vi "GetCurrentPosition.vi"(8 "error in (no error)":errorcluster, 11 "Serial Controller in":refnum<class "Serial Controller.lvclass">) -> (0 "error out":errorcluster, 1 "PositionBundle":cluster{"X":dbl, "Y":dbl, "Z":dbl, "Depth":dbl}, 2 "Position":dbl[](array[numeric]), 3 "Serial Controller out":refnum<class "Serial Controller.lvclass">)   [LabVIEW 2012, in "Serial Controller.lvclass"]
uses:
  Serial Controller.lvclass
  Serial Controller.lvclass/Serial Controller.ctl
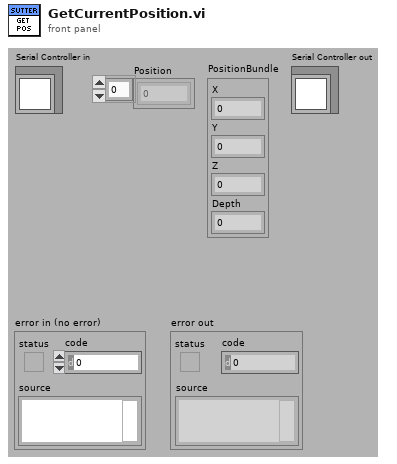
[diagram p1: front panel]
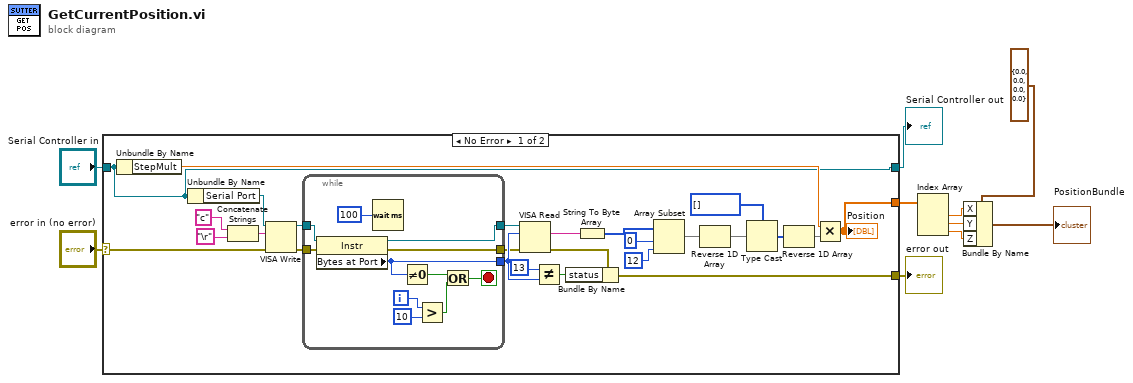
[diagram p0: block diagram]
diagram:
  n1 = case shown="No Error" "error in (no error)" {
    selector: "error in (no error)" -> [w16 w49]
    tunnel: [w12 w49] -> w3
    tunnel: [w26 w48] -> w9
    tunnel: "Serial Controller in" -> [w26 w48]
    tunnel: [w27 _] -> w7
    frame No Error {
      n2 = Unbundle By Name(w26) -> ("StepMult"=w28:dbl)
      n3 = Unbundle By Name(w26) -> ("Serial Port"=w20:refnum<visa-resource-name>)
      n4 = Concatenate Strings("c" ("string"), "\r" ("write buffer")) -> (w17:string)
      n5 = VISA Write(VISA resource name=w20, write buffer=w17, error in (no error)=w16) -> (VISA resource name out=w21:refnum<visa-resource-name>, error out=w15:errorcluster)  [unwired: 1 out]
      n6 = while {
        tunnel: w21 -> [w47]
        tunnel: w15 -> [w46]
        tunnel: [w45] -> w25
        tunnel: [w41] -> w24
        tunnel: [w40] -> w14
        i -> [w39]
        stop <- w43 stop-if-true
        n7 = property class="Instr"(reference=w47, error in=w46) -> (reference out=w45:refnum<visa-resource-name>, error out=w40:errorcluster, "Bytes at Port"=w41:u32)
        n8 = Wait (ms)(milliseconds to wait=u32 100) -> ()  [unwired: 1 out]
        n9 = Not Equal To 0?(x=w41) -> (x != 0?=w42:bool)
        n10 = Greater?(x=w39, y=10) -> (0:w37:bool)
        n11 = Or(x=w42, y=w37) -> (x .or. y?=w43:bool)
      }
      n12 = VISA Read(VISA resource name=w25, byte count=w24, error in (no error)=w14) -> (read buffer=w22:string, error out=w13:errorcluster)  [unwired: 2 out]
      n13 = Not Equal?(x=u32 13, y=w24) -> (x != y?=w11:bool)
      n14 = Bundle By Name(cluster=w13, "status"=w11) -> (w12:errorcluster)
      n15 = String To Byte Array(string=w22) -> (unsigned byte array=w36:u8[])
      n16 = Array Subset(array=w36, index=0, length=12) -> (w32:u8[])
      n17 = Reverse 1D Array(array=w32) -> (reversed array=w31:u8[])
      n18 = Type Cast(type=i32[] [], x=w31) -> (*(type *) &x=w30:i32[])
      n19 = Reverse 1D Array(array=w30) -> (reversed array=w29:i32[])
      n20 = Multiply(x=w28, y=w29) -> (x*y=w27:dbl[])
      "Position" <- w27
    }
    frame Error {
    }
  }
  "error out" <- w3
  "Serial Controller out" <- w9
  n21 = Index Array(array=w7) -> (element #1=w6:dbl, element #2=w5:dbl, element #3=w4:dbl)  [unwired: 3 in]
  n22 = Bundle By Name(cluster=cluster{"X":dbl, "Y":dbl, "Z":dbl, "Depth":dbl} {"X"=0.0, "Y"=0.0, "Z"=0.0, "Depth"=0.0} ("Cluster"), "X"=w6, "Y"=w5, "Z"=w4) -> (→"PositionBundle":cluster{"X":dbl, "Y":dbl, "Z":dbl, "Depth":dbl})
